vi "Output Enable Read Single.vi"() -> ()   [LabVIEW 2023, in "Output Enable.lvclass"]
uses:
  Output Enable.lvclass
  Output Enable.lvclass/Output Enable.ctl
  <vilib>/ADAS Replay HIL/Channels/Tag Wrapper/Tag Wrapper.lvlib
  8214ba14-0da7-445b-a3d2-4f374d612fdf.vi
  <vilib>/ADAS Replay HIL/Channels/Tag Wrapper/Polymorphic/Read Channel (Boolean).vi
panel:
  out "Output Enable out":refnum<class "Output Enable.lvclass">
  out "OE Out":bool
  in  "Output Enable in":refnum<class "Output Enable.lvclass">
  in  "Channel Index":i32=1
  out "Changed or First Call?":bool
  out "error out":errorcluster
  in  "error in":errorcluster
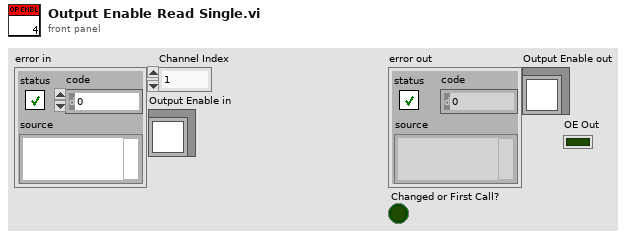
[diagram p1: front panel]
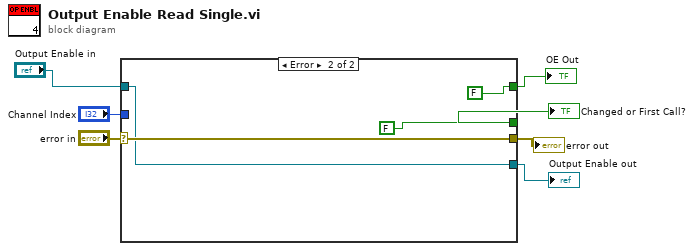
[diagram p0: block diagram]
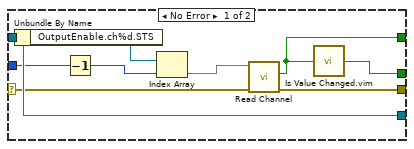
[diagram p2: hidden frame]
diagram:
  n1 = case shown="Error" "error in" {
    selector: "error in" -> [w14 w20]
    tunnel: [w13 w20] -> w6
    tunnel: [w16 w19] -> w1
    tunnel: "Output Enable in" -> [w16 w19]
    tunnel: [w12 FALSE ("Value out")] -> w2
    tunnel: [w11 FALSE ("changed or first call?")] -> w5
    tunnel: "Channel Index" -> [w10 _]
    frame No Error {
      n2 = Unbundle By Name(w16) -> ("OutputEnable.ch%d.STS"=w15:refnum<k21>)
      n3 = Decrement(x=w10) -> (x-1=w9:i32)
      n4 = Index Array(array=w15, index=w9) -> (element=w8)
      n5 = call-poly <vilib>:"Read Channel.vi"("error in"=w14, "ADAS HIL Channel in"=w8) -> ("error out"=w13:errorcluster, "Value out"=w12:bool)  [unwired: 6 in, 2 out]
      n6 = call "Is Value Changed.vim"("value"=w12) -> ("changed or first call?"=w11:bool)
    }
    frame Error {
    }
  }
  "error out" <- w6
  "Changed or First Call?" <- w5
  "OE Out" <- w2
  "Output Enable out" <- w1
